vi "Ex5.vi"() -> ()   [LabVIEW 2012]
uses:
  <userlib>/ROSforLV/ROS/Code/SubVIs/BaxterCamera.ctl
panel:
  in  "stop":bool
  out "image":picture
  out "Cameras List":T1={"Number of Cameras"=3, "Cameras"=["head_camera", "left_hand_camera", "right_hand_camera"], "OK Byte"=0}
  in  "Camera Settings":T3={"Camera"=enum."left_hand_camera", "FPS"=20.0, "Camera Controls"=[{"id"=0, "value"=0}], "Resolution"=enum."(320, 200)"}
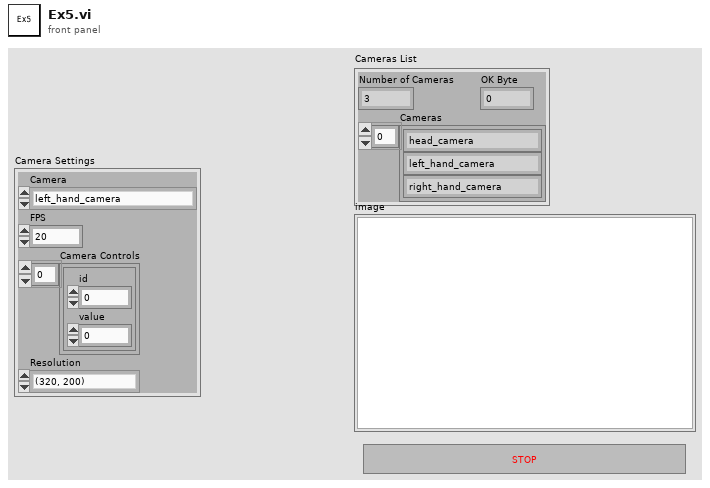
[diagram p1: front panel]
types:
  T1 = cluster{"Number of Cameras":i32, "Cameras":string[], "OK Byte":u8}
  T2 = typedef "BaxterCamera.ctl" = enum16{"left_hand_camera", "right_hand_camera", "head_camera"}
  T3 = cluster{"Camera":T2, "FPS":sgl, "Camera Controls":cluster{"id":i32, "value":i32}[], "Resolution":enum16{"(1280, 800)", "(960, 600)", "(640, 400)", "(480, 300)", "(384, 240)", "(320, 200)"}}
  T4 = typedef "imagedata.ctl" = cluster{"image type":i32, "image depth":i32, "image":u8[], "mask":u8[], "colors":u32[], "Rectangle":cluster{"left":i16, "top":i16, "right":i16, "bottom":i16}}
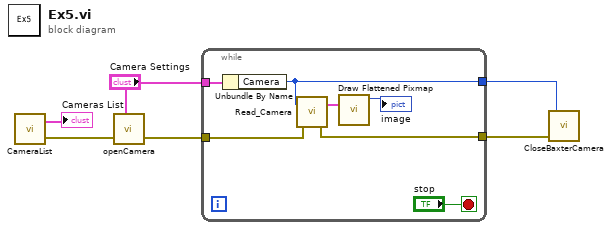
[diagram p0: block diagram]
diagram:
  n1 = call <userlib>:"CameraList.vi"() -> ("error out"=w6:errorcluster, "Cameras List"=→"Cameras List":T1)  [unwired: 2 in]
  n2 = call <userlib>:"openCamera.vi"("error in"=w6, "Camera Settings"="Camera Settings") -> ("error out"=w4:errorcluster)  [unwired: 1 in, 1 out]
  n3 = while {
    tunnel: w4 -> [w13]
    tunnel: [w12] -> w3
    tunnel: [w8] -> w2
    tunnel: "Camera Settings" -> [w7]
    stop <- "stop" stop-if-true
    n4 = Unbundle By Name(w7) -> ("Camera"=w8:T2)
    n5 = call <userlib>:"Read_Camera.vi"("error in"=w13, "Camera"=w8) -> ("error out"=w12:errorcluster, "image data"=w10:T4)  [unwired: 1 in]
    n6 = call <vilib>:"Draw Flattened Pixmap.vi"("image data"=w10) -> ("new picture"=→"image":picture)  [unwired: 8 in]
  }
  n7 = call <userlib>:"CloseBaxterCamera.vi"("error in"=w3, "Camera"=w2) -> ()  [unwired: 1 in, 3 out]
